vi "LM model function and gradient (1-Exp, Convolved, Periodic) v3.vi"(3 "output control":T1, 4 "data":variant, 5 "X":dbl[](array[numeric]), 6 "a":dbl[](array[numeric]) format="%_5g") -> (0 "error out":errorcluster, 1 "f'(X,a)":dbl[][](array[numeric]), 2 "f(X,a)":dbl[](array[numeric]))   [LabVIEW 2021, in "Fits.lvlib"]
doc: "This template is the starting point for creating a model function to be passed to the Nonlinear Curve Fit.vi."
uses:
  Fits.lvlib
  <vilib>/gmath/NumericalOptimization/LM_output select.ctl
  1-Exp Parameters.ctl
  Fit Control Data.ctl
  Graphs/XY Graph/XY Plot Data.ctl
  9edc71ac-b7a9-4893-b72d-f95f6606a6ac.vi
  Graphs/XY Graph/XY Graph Add-Ons.lvlib
  <vilib>/gmath/NI_Gmath.lvlib
panel:
  # "t0\n\nBL\n\nA1\n\ntau1"
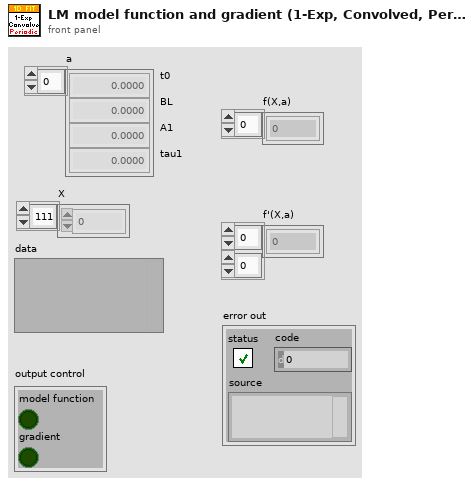
[diagram p1: front panel]
types:
  T1 = typedef "NI_Gmath.lvlib/LM_output select.ctl" = cluster{"model function":bool, "gradient":bool}
  T2 = typedef "Fits.lvlib/1-Exp Parameters.ctl" = cluster{"t_0":dbl, "B":dbl, "A":dbl, "tau":dbl, "T":dbl, "sigma":dbl}
  T3 = typedef "Fits.lvlib/Fit Control Data.ctl" = cluster{"IRF":T4, "Laser Period":dbl, "SYNC Period":dbl}
  T4 = typedef "XY Graph Add-Ons.lvlib/XY Plot Data.ctl" = cluster{"X Array":dbl[], "Y Array":dbl[]}
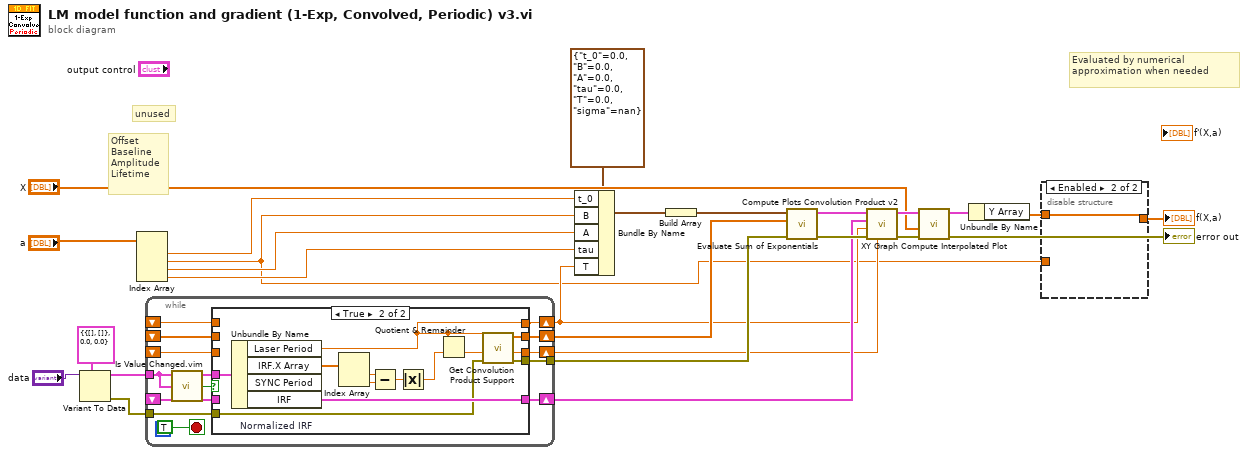
[diagram p0: block diagram]
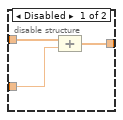
[diagram p2: hidden frame]
diagram:
  # "unused"
  # "Evaluated by numerical approximation when needed"
  # "Offset\nBaseline\nAmplitude\nLifetime"
  n1 = Variant To Data(type=T3 {"IRF"={"X Array"=[], "Y Array"=[]}, "Laser Period"=0.0, "SYNC Period"=0.0} ("Fit Control Data"), Variant="data") -> (data=w24:T3, error out=w14:errorcluster)  [unwired: 1 in]
  n2 = Index Array(array="a") -> (element #1=w18:dbl, element #2=w1:dbl, element #3=w17:dbl, element #4=w21:dbl)  [unwired: 4 in]
  n3 = while {
    tunnel: w24 -> [w35]
    tunnel: w14 -> [w38]
    tunnel: [w37] -> w13
    shift-right: [w36] -> w12
    shift-left: _ -> [w32]
    shift-right: [w39] -> w4
    shift-left: _ -> [w31]
    shift-right: [w30] -> w3
    shift-left: _ -> [w29]
    shift-right: [w28] -> w2
    shift-left: _ -> [w27]
    stop <- TRUE stop-if-true
    n4 = call "Is Value Changed.vim"("value"=w35) -> ("changed or first call?"=w33:bool)
    n5 = case shown="True" w33 {
      tunnel: [w42 w57] -> w39
      tunnel: w38 -> [w43 w50]
      tunnel: [w43 w49] -> w37
      tunnel: [w44 w48] -> w36
      tunnel: w35 -> [_ w47]
      tunnel: w32 -> [w44 _]
      tunnel: w31 -> [w42 _]
      tunnel: [w41 w46] -> w30
      tunnel: w29 -> [w41 _]
      tunnel: [w40 w45] -> w28
      tunnel: w27 -> [w40 _]
      frame False {
      }
      frame True {
        n6 = Unbundle By Name "Normalized IRF"(w47) -> ("Laser Period"=w46:dbl, "IRF.X Array"=w56:dbl[], "IRF"=w57:T4)  [unwired: 1 out]
        n7 = Index Array(array=w56) -> (element #1=w55:dbl, element #2=w54:dbl)  [unwired: 2 in]
        n8 = Subtract(x=w55, y=w54) -> (x-y=w53:dbl)
        n9 = Absolute Value(x=w53) -> (abs(x)=w52:dbl)
        n10 = Quotient & Remainder(x=w46, y=w52) -> (floor(x/y)=w51:dbl)  [unwired: 1 out]
        n11 = call "Get Convolution Product Support.vi"("Error In"=w50, "# Values"=w51, "IRF Period"=w46) -> ("Error Out"=w49:errorcluster, "Step"=w45:dbl, "Ramp"=w48:dbl[])  [unwired: 6 in]
      }
    }
  }
  n12 = Bundle By Name(cluster=T2 {"t_0"=0.0, "B"=0.0, "A"=0.0, "tau"=0.0, "T"=0.0, "sigma"=nan} ("Gate & Decay Parameters"), "t_0"=w18, "B"=w1, "A"=w17, "tau"=w21, "T"=w3) -> (w22:T2)
  n13 = Build Array(w22) -> (w19:T2[])
  n14 = call "Evaluate Sum of Exponentials.vi"("error in (no error)"=w13, "Ramp"=w12, "Exp Parameters Array"=w19) -> ("error out"=w15:errorcluster, "Plot"=w5:T4)  [unwired: 7 in]
  n15 = call "Compute Plots Convolution Product v2.vi"("Step"=w2, "Error In"=w15, "Period"=w3, "Plot 2 (kernel)"=w4, "Plot 1 (function)"=w5) -> ("Error Out"=w9:errorcluster, "Convolution Product"=w11:T4)  [unwired: 4 in, 1 out]
  n16 = call "XY Graph Compute Interpolated Plot.vi"("Error In"=w9, "Ramp"="X", "Plot"=w11) -> ("Error Out"=→"error out":errorcluster, "Interpolated Plot"=w10:T4)  [unwired: 7 in]
  n17 = Unbundle By Name(w10) -> ("Y Array"=w16:dbl[])
  n18 = disable-structure shown="Enabled" {
    disable-tunnel: [w60 w61] -> w20
    disable-tunnel: w16 -> [w59 w61]
    disable-tunnel: w1 -> [w58 _]
    frame Disabled {
      n19 = Compound Arithmetic op=ADD(w59, w58) -> (w60:dbl[])
    }
    frame Enabled {
    }
  }
  "f(X,a)" <- w20
